vi "Create.vi"(8 "error in (no error)":errorcluster, 10 "Expected":T1) -> (0 "error out":errorcluster, 3 "IsType":refnum<class "IsType.lvclass">)   [LabVIEW 2017, in "Transparent Assertions.lvlib" / "Constraints.lvlib" / "IsType.lvclass"]
uses:
  IsType.lvclass
  <vilib>/Utility/Data Type/Type Definitions/Data Type.ctl
  IsType.lvclass/IsType.ctl
  <vilib>/Utility/Data Type/NI_Data Type.lvlib
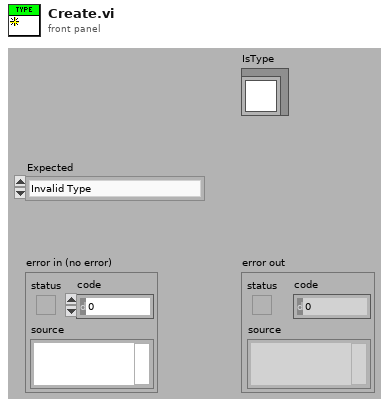
[diagram p1: front panel]
types:
  T1 = typedef "NI_Data Type.lvlib/Data Type.ctl" = enum8{"Invalid Type", "Void", "I8", "I16", "I32", "I64", "U8", "U16", "U32", "U64", "Single Float", "Double Float", "Extended Float", "Single Complex", "Double Complex", "Extended Complex", "Enum U8", "Enum U16", "Enum U32", "Enum U64", "Single Float With Unit", "Double Float With Unit", "Extended Float With Unit", "Single Complex with Unit", "Double Complex with Unit", "Extended Complex with Unit", "Boolean", "String", "Path", "Picture", "Tag", "Array", "Cluster", "Variant", "LV Variant", "Waveform", "Timestamp", "Digital Waveform", "Digital Data", "ExpressData", "Refnum", "External Data", "VI", "Poly VI", "LabVIEW Class Instance", "Fixed Point"}
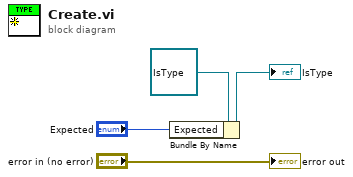
[diagram p0: block diagram]
diagram:
  n1 = Bundle By Name(cluster=refnum<class "IsType.lvclass"> refnum ("IsType"), "Expected"="Expected") -> (→"IsType":refnum<class "IsType.lvclass">)
  "error out" <- "error in (no error)"
